vi "Data_Graph_Stat_Meteo.vi"(1 "mesure cherchée":string, 2 "Chaine Arduino":string) -> (0 "Numeric":dbl)   [LabVIEW 2018]
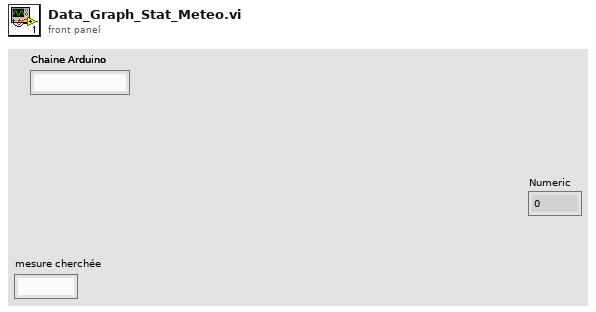
[diagram p1: front panel]
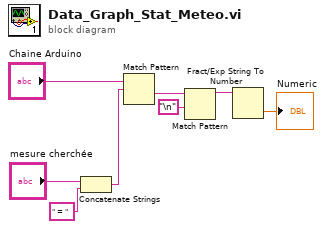
[diagram p0: block diagram]
diagram:
  n1 = Concatenate Strings("mesure cherchée", " = " ("string")) -> (w6:string)
  n2 = Match Pattern(string="Chaine Arduino", regular expression=w6) -> (after substring=w4:string)  [unwired: 1 in, 3 out]
  n3 = Match Pattern(string=w4, regular expression="\n") -> (before substring=w2:string)  [unwired: 1 in, 3 out]
  n4 = Fract/Exp String To Number(string=w2) -> (number=→"Numeric":dbl)  [unwired: 3 in, 1 out]
